vi "RP IV analysis.vi"() -> ()   [LabVIEW 2016]
uses:
  Waform generation/I-V parameters.ctl
panel:
  in  "Slicing threshold":dbl format="%#_6p"
  in  "Preamp\nsetting I":dbl=100.0 format="x%#_6p"
  in  "Preamp\nsetting V":dbl=100.0 format="x%#_6p"
  in  "Invert V":bool
  in  "Invert I":bool
  out "Iv curves":T1(graph)
  out "Current vs Time":dbl[](graph)
  in  "Current Channel":string="CH1"
  out "Voltage vs Time":dbl[](graph)
  in  "I-V parameters":T2={"Start magnitude"=0.01, "Magnitude increment"=0.001, "Number of pulses"=8, "Baseline length"=224, "Ramp length"=32, "Top  length"=224, "Threshold "=1e-05, "Processing Delay"=126, "Valhalla range"=0.001, "Interpolation"=64} {"Valhalla range" format="%#_6pA"; "Processing Delay" format="%dpts"; "Threshold" format="%#_6pV"; "Top  length" format="%dpts"; "Ramp length" format="%dpts"; "Baseline length" format="%dpts"; "Magnitude increment" format="%#_6pA"; "Start magnitude" format="%#_6pA"}
  in  "Voltage Channel":string="CH0"
  in  "Delay":dbl=0.013735 format="%#_6p"
  in  "File Path":path
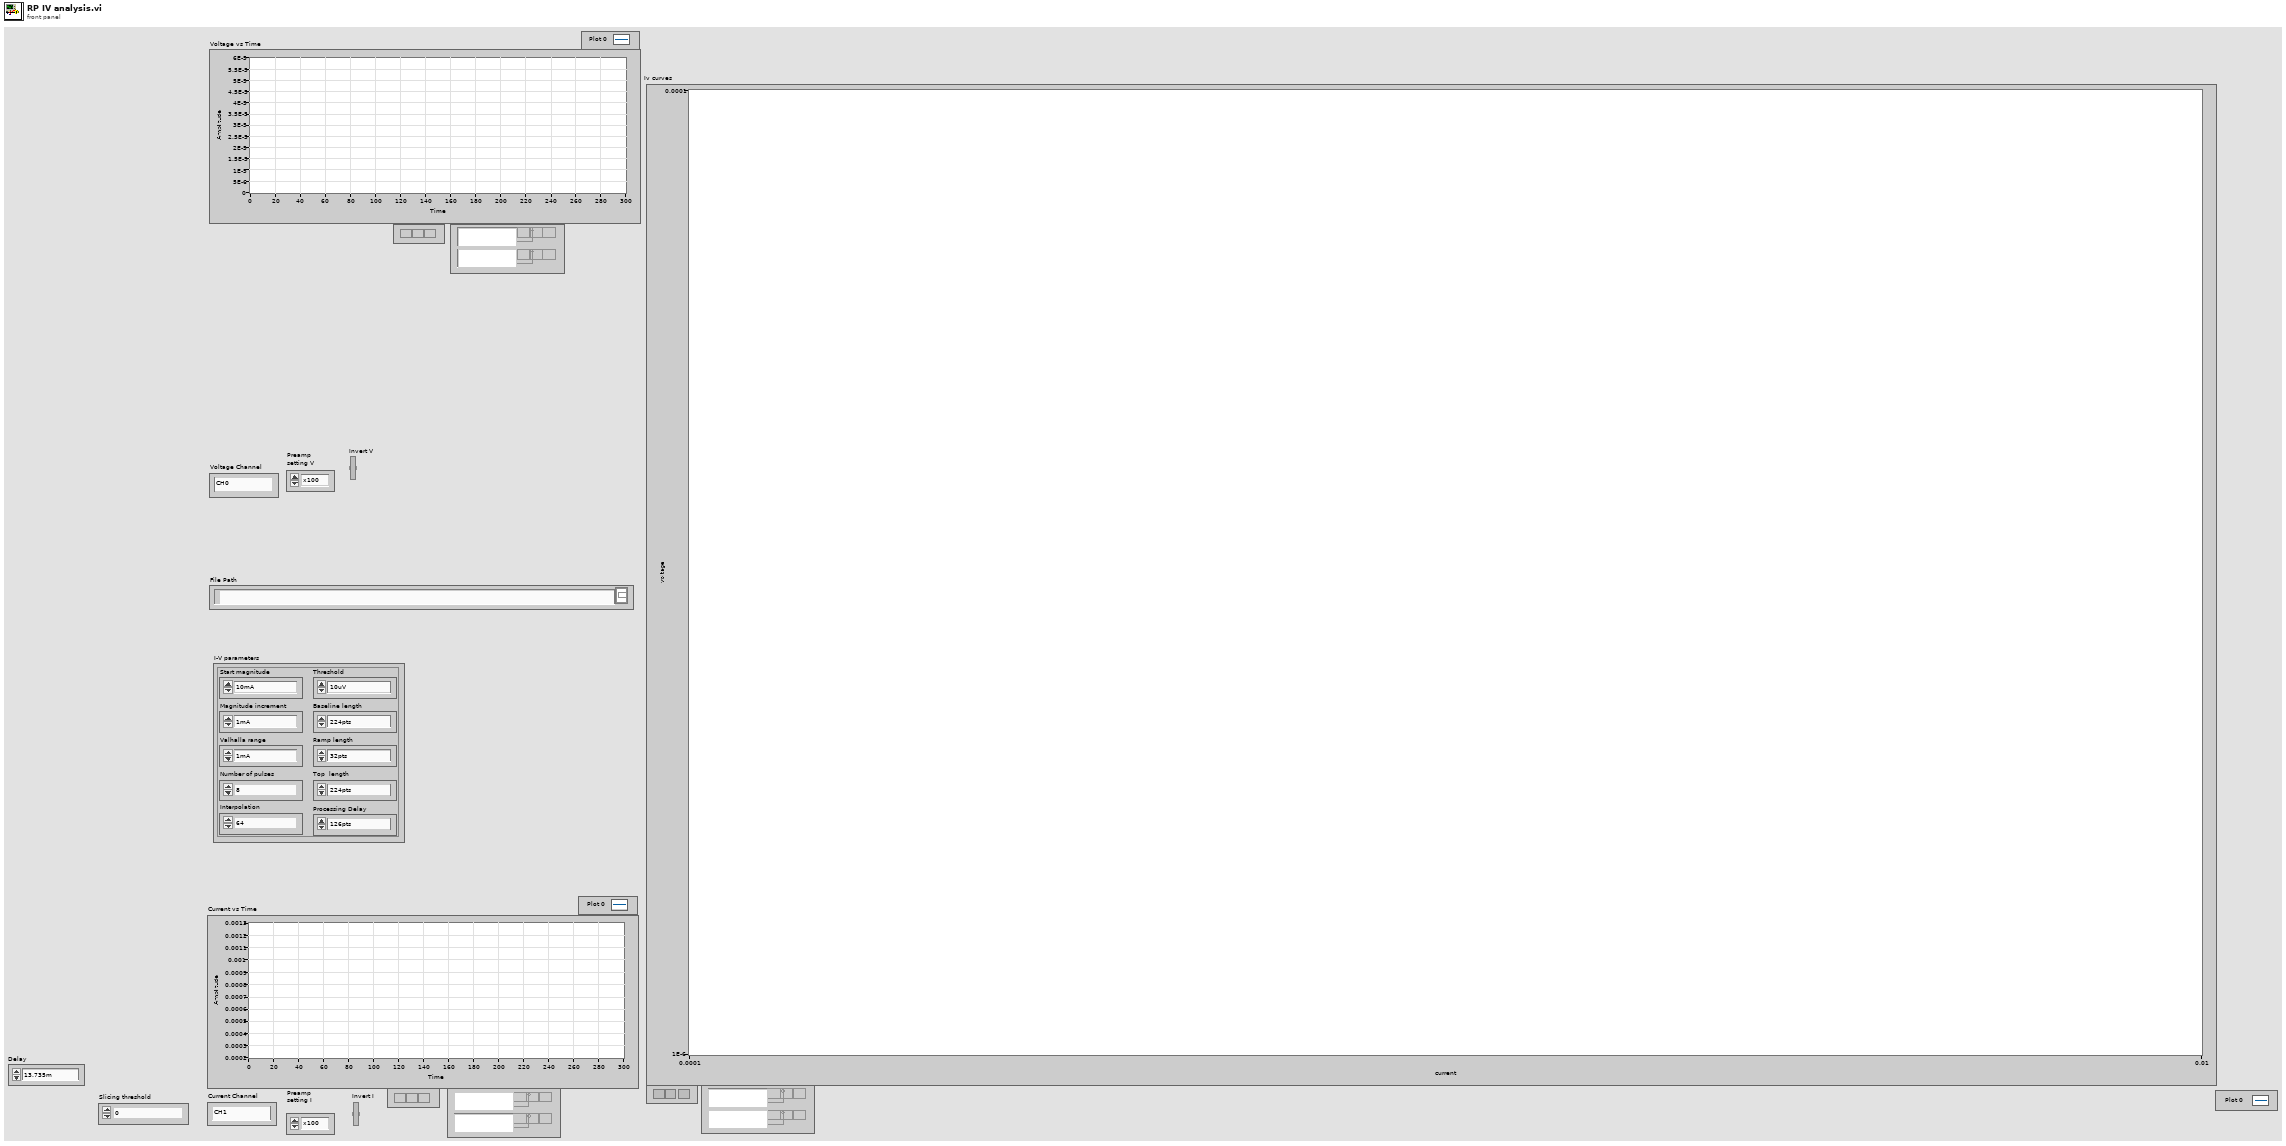
[diagram p1: front panel]
types:
  T1 = cluster{"Sliced array":dbl[], "Sliced array":dbl[]}[]
  T2 = typedef "I-V parameters.ctl" = cluster{"Start magnitude":dbl, "Magnitude increment":dbl, "Number of pulses":i32, "Baseline length":i32, "Ramp length":i32, "Top  length":i32, "Threshold ":dbl, "Processing Delay":u16, "Valhalla range":dbl, "Interpolation":i32}
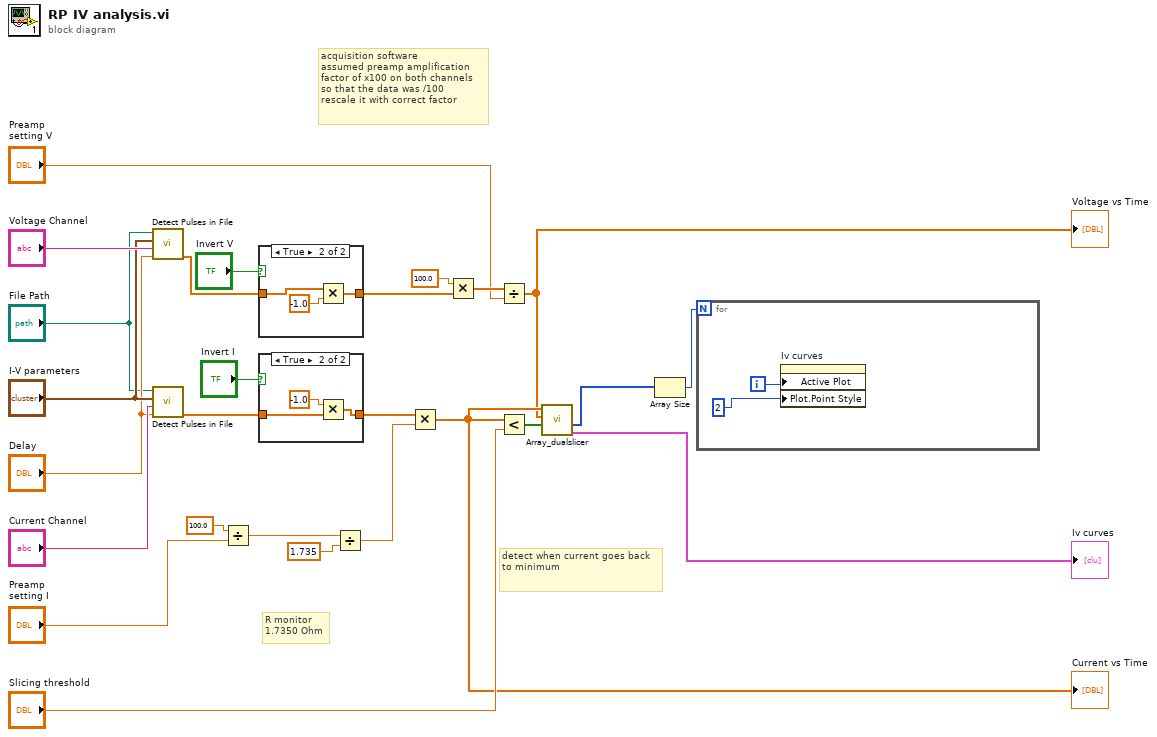
[diagram p0: block diagram]
diagram:
  # "detect when current goes back to minimum"
  # "R monitor\n1.7350 Ohm"
  # "acquisition software\nassumed preamp amplification\nfactor of x100 on both channels\nso that the data was /100\nrescale it with correct factor"
  n1 = call "Detect Pulses in File.vi"("Delay"="Delay", "Channel name"="Voltage Channel", "I-V parameters"="I-V parameters", "File Path"="File Path") -> ("Avg signal minus\nAvg background"=w19:dbl[])  [unwired: 5 in, 2 out]
  n2 = call "Detect Pulses in File.vi"("Delay"="Delay", "Channel name"="Current Channel", "I-V parameters"="I-V parameters", "File Path"="File Path") -> ("Avg signal minus\nAvg background"=w14:dbl[])  [unwired: 5 in, 2 out]
  n3 = Divide(x=100.0, y="Preamp\nsetting I") -> (x/y=w12:dbl)
  n4 = case shown="True" "Invert V" {
    tunnel: w19 -> [w27 w30]
    tunnel: [w27 w28] -> w15
    frame False {
    }
    frame True {
      n5 = Multiply(x=w30, y=-1.0) -> (x*y=w28:dbl[])
    }
  }
  n6 = case shown="True" "Invert I" {
    tunnel: [w31 w33] -> w9
    tunnel: w14 -> [w31 w32]
    frame False {
    }
    frame True {
      n7 = Multiply(x=-1.0, y=w32) -> (x*y=w33:dbl[])
    }
  }
  n8 = Divide(x=w12, y=1.735) -> (x/y=w10:dbl)
  n9 = Multiply(x=w9, y=w10) -> (x*y=w6:dbl[])
  "Current vs Time" <- w6
  n10 = Multiply(x=100.0, y=w15) -> (x*y=w18:dbl[])
  n11 = Divide(x=w18, y="Preamp\nsetting V") -> (x/y=w5:dbl[])
  "Voltage vs Time" <- w5
  n12 = Less?(x=w6, y="Slicing threshold") -> (x < y?=w4:bool[])
  n13 = call "Array_dualslicer.vi"("X array"=w6, "Y array"=w5, "Slicing array"=w4) -> ("Lengths"=w2:i32[], "Output cluster"=→"Iv curves":cluster{dbl[], dbl[]}[])  [unwired: 1 in, 4 out]
  n14 = Array Size(array=w2) -> (size(s)=w1:i32)
  n15 = for {
    N: w1 -> [_]
    i -> [w36]
    n16 = property on="Iv curves" class="XYGraph (strict)"("Active Plot"=w36, "Plot.Point Style"=u8 2) -> ()  [unwired: 2 in, 2 out]
  }
